vi "Tip String Write.vi"(4 "error in (no error)":errorcluster, 5 "Value":string, 6 "Container State":T3, 7 "Display State In":T1={"Buttons Displayed"=0, "Button States"=[], "Button Size"=0, "Button Style"=enum."Classic", "Active Button"=0, "Force Regen?"=FALSE, "Tip String Ref"=refnum}) -> (0 "error out":errorcluster, 3 "Display State Out":T1={"Buttons Displayed"=0, "Button States"=[], "Button Size"=0, "Button Style"=enum."Classic", "Active Button"=0, "Force Regen?"=FALSE, "Tip String Ref"=refnum})   [LabVIEW 2012, in "Toolbar.xctl"]
doc: "The toolabr can post status messages back to a user supplied string indicator reference. This sets that string value."
uses:
  Toolbar.xctl
  <vilib>/_xctls/Container State.ctl
  Toolbar State.ctl
  Button_Class/Button.lvclass
  Button_Class/Type Defs/Button Style.ctl
  <vilib>/_xctls/XControlSupport.lvlib
panel:
  # "Replace the Value Control below with a Control of desired type.\nDo not remove this Control or the others from the connector pane.\nDo not change the connector pane pattern.\nThe Value control should always be the third terminal from top on the input side in the connector pane."
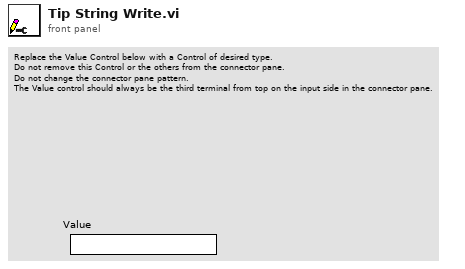
[diagram p1: front panel]
types:
  T1 = typedef "Toolbar.xctl/Toolbar State.ctl" = cluster{"Buttons Displayed":i32, "Button States":refnum<class "Button.lvclass">[], "Button Size":i32, "Button Style":T2, "Active Button":i32, "Force Regen?":bool, "Tip String Ref":refnum<vi>}
  T2 = typedef "Button.lvclass/Button Style.ctl" = enum16{"System", "Modern", "Classic", "Rounded", "Silver", "Ni Theme", "Metallic"}
  T3 = typedef "XControlSupport.lvlib/Container State.ctl" = cluster{"Indicator?":bool, "Run Mode?":bool, " Refnum":refnum<vi>}
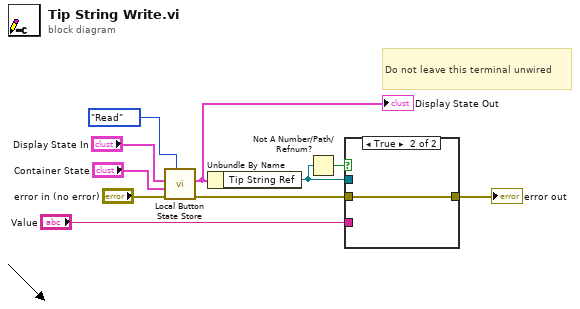
[diagram p0: block diagram]
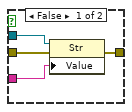
[diagram p2: hidden frame]
diagram:
  # "Do not leave this terminal unwired"
  n1 = call "Local Button State Store.vi"("Operation"=enum16{"Read", "Write"}."Read", "error in (no error)"="error in (no error)", "Container State"="Container State", "Display State In"="Display State In") -> ("error out"=w3:errorcluster, "Display State Out"=w2:T1)  [unwired: 6 out]
  "Display State Out" <- w2
  n2 = Unbundle By Name(w2) -> ("Tip String Ref"=w9:refnum<vi>)
  n3 = Not A Number/Path/Refnum?(number/path/refnum=w9) -> (NaN/Path/Refnum?=w10:bool)
  n4 = case shown="True" w10 {
    tunnel: w9 -> [w14 _]
    tunnel: "Value" -> [w13 _]
    tunnel: w3 -> [w12 w15]
    tunnel: [w11 w15] -> w7
    frame False {
      n5 = property class="Str"(reference=w14, error in=w12, "Value"=w13) -> (error out=w11:errorcluster)  [unwired: 1 out]
    }
    frame True {
    }
  }
  "error out" <- w7
